vi "PathPlanner_PathFinder_DoMinor.vi"   [LabVIEW 2019, in "PathPlanner24.lvlib"]
uses:
  PathPlanner24.lvlib
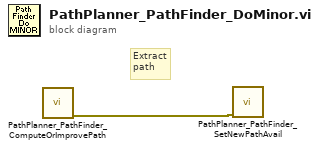
[diagram p0: block diagram]
diagram:
  # "Extract\npath"
  n1 = call "PathPlanner_PathFinder_ComputeOrImprovePath.vi"() -> ("error out"=w1:errorcluster)  [unwired: 11 in]
  n2 = call "PathPlanner_PathFinder_SetNewPathAvail.vi"("error in (no error)"=w1) -> ()  [unwired: 10 in, 1 out]
